vi "ep_Valid Speed Range.vi"(8 "speed range ratio":dbl=0.2, 9 "nameplate information":T1, 10 "speed [RPM]":dbl, 11 "fundamental frequency [Hz]":dbl) -> (2 "trigger?":bool, 3 "speed range [RPM]":cluster{"sync speed":dbl, "full load speed":dbl})   [LabVIEW 2017]
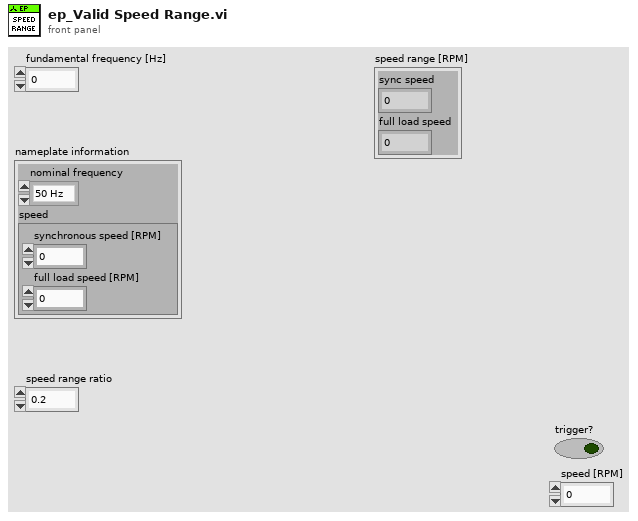
[diagram p1: front panel]
types:
  T1 = cluster{"nominal frequency":enum16{"50 Hz", "60 Hz"}, "speed":cluster{"synchronous speed [RPM]":dbl, "full load speed [RPM]":dbl}}
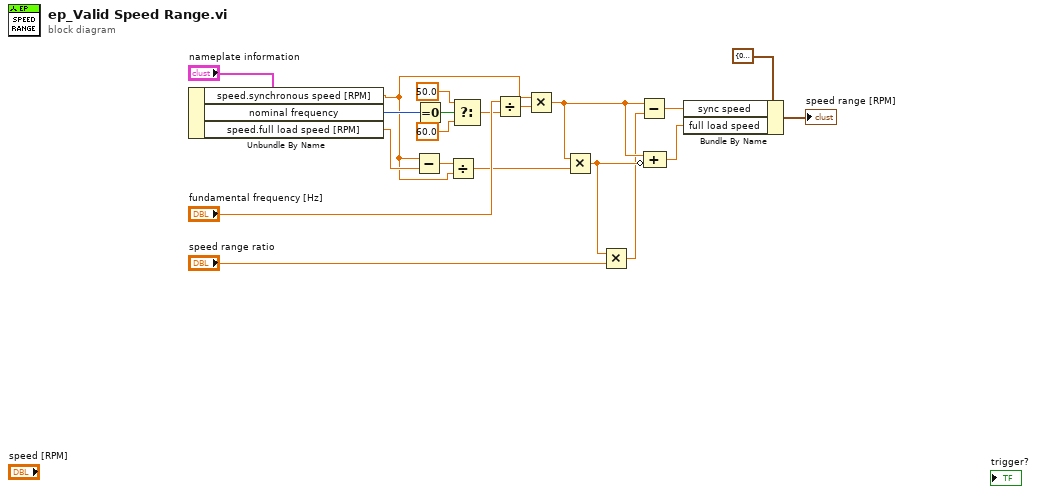
[diagram p0: block diagram]
diagram:
  n1 = Unbundle By Name("nameplate information") -> ("speed.synchronous speed [RPM]"=w10:dbl, "nominal frequency"=w12:enum16{"50 Hz", "60 Hz"}, "speed.full load speed [RPM]"=w18:dbl)
  n2 = Subtract(x=w10, y=w18) -> (x-y=w11:dbl)
  n3 = Equal To 0?(x=w12) -> (x = 0?=w13:bool)
  n4 = Divide(x=w11, y=w10) -> (x/y=w9:dbl)
  n5 = Select(t=50.0, s=w13, f=60.0) -> (s? t:f=w15:dbl)
  n6 = Divide(x="fundamental frequency [Hz]", y=w15) -> (x/y=w16:dbl)
  n7 = Multiply(x=w10, y=w16) -> (x*y=w4:dbl)
  n8 = Multiply(x=w4, y=w9) -> (x*y=w3:dbl)
  n9 = Multiply(x=w3, y="speed range ratio") -> (x*y=w1:dbl)
  n10 = Subtract(x=w4, y=w1) -> (x-y=w5:dbl)
  n11 = Compound Arithmetic op=ADD(w4, invert w3) -> (w2:dbl)
  n12 = Bundle By Name(cluster=cluster{"sync speed":dbl, "full load speed":dbl} {"sync speed"=0.0, "full load speed"=0.0} ("measured speed [RPM]"), "sync speed"=w5, "full load speed"=w2) -> (→"speed range [RPM]":cluster{"sync speed":dbl, "full load speed":dbl})
